vi "EventCallBack.vi"(4 "?":refnum<vi>, 5 "Event Data":cluster{"FrameNumber":i32}, 6 "Control Ref":refnum<k7>, 7 "Event Common Data":T1) -> ()   [LabVIEW 2010]
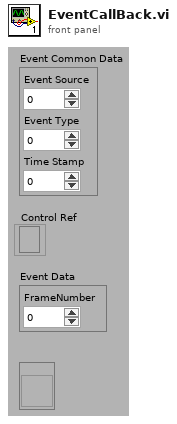
[diagram p1: front panel]
types:
  T1 = cluster{"Event Source":i32, "Event Type":u32, "Time Stamp":u32}
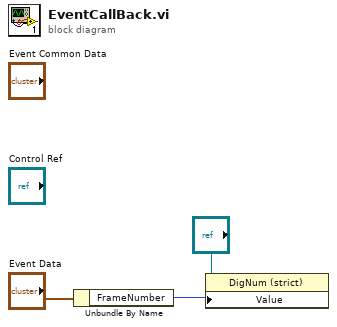
[diagram p0: block diagram]
diagram:
  n1 = Unbundle By Name("Event Data") -> ("FrameNumber"=w1:i32)
  n2 = property class="DigNum (strict)"(reference="?", "Value"=w1) -> ()  [unwired: 1 in, 2 out]
